vi "Generate Class and Subclasses.vi"(7 "Owning LVLib":refnum<vi>, 8 "Class Ref Map":T1, 9 "Class Name":string, 10 "Inheritance Map":T1, 11 "Base Class":refnum<vi>) -> (0 "Augmented Class Ref Map":T1, 2 "Reduced Inheritance Map":T1, 3 "Base Class Dup":refnum<vi>)   [LabVIEW 2013]
uses:
  <userlib>/ICON Technologies/ICON Maps/lvlib/Map.ctl
  <userlib>/ICON Technologies/ICON Maps/lvlib/_Polymorphic Instances/Map_Insert_Variant.vi
  <userlib>/ICON Technologies/ICON Maps/ICON Maps.lvlib
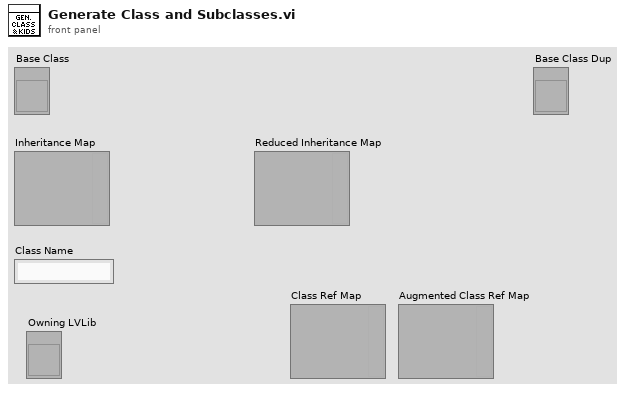
[diagram p1: front panel]
types:
  T1 = typedef "ICON Maps.lvlib/Map.ctl" = variant
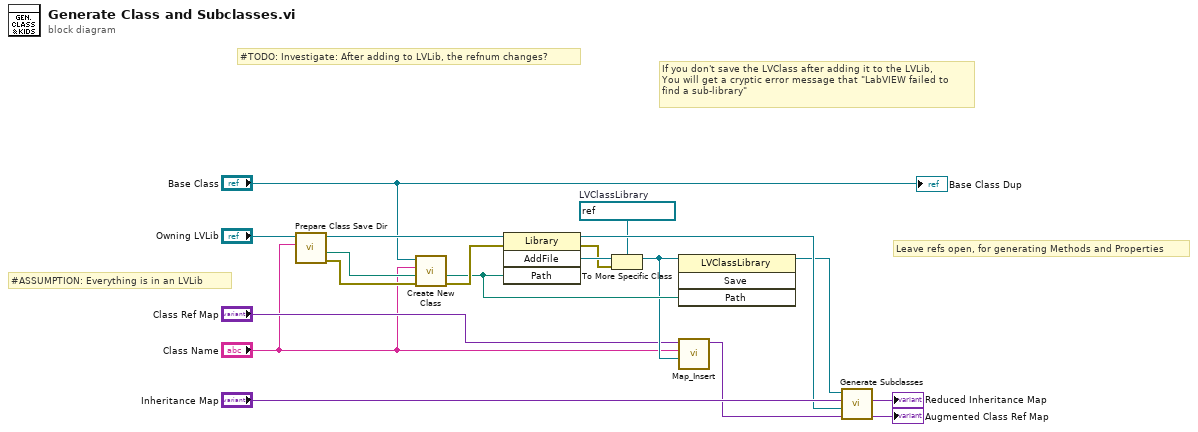
[diagram p0: block diagram]
diagram:
  w11 = refnum<vi> refnum  # LVClassLibrary
  # "Leave refs open, for generating Methods and Properties"
  # "#ASSUMPTION: Everything is in an LVLib"
  # "If you don't save the LVClass after adding it to the LVLib,\nYou will get a cryptic error message that \"LabVIEW failed to\nfind a sub-library\""
  # "#TODO: Investigate: After adding to LVLib, the refnum changes?"
  n1 = call "Prepare Class Save Dir.vi"("Class Name"="Class Name", "Owning LVLib"="Owning LVLib") -> ("Error Out"=w13:errorcluster, "Class Path"=w8:path, "Owning LVLib Dup"=w9:refnum<vi>)  [unwired: 7 in]
  n2 = call "Create New Class.vi"("Error In"=w13, "Class Path"=w8, "Class Name"="Class Name", "Base Class"="Base Class") -> ("Error Out"=w12:errorcluster, "Class Path Dup"=w7:path)  [unwired: 5 in, 1 out]
  n3 = invoke class="Library" method="AddFile"(reference=w9, error in=w12, "Path"=w7) -> (reference out=w16:refnum<vi>, error out=w14:errorcluster, "AddFile"=w17:refnum<vi>)  [unwired: 1 in, 1 out]
  n4 = To More Specific Class(target class=w11, reference=w17, error in=w14) -> (specific class reference=w6:refnum<vi>)  [unwired: 1 out]
  n5 = invoke class="LVClassLibrary" method="Save"(reference=w6, "Path"=w7) -> (reference out=w15:refnum<vi>)  [unwired: 2 in, 3 out]
  n6 = call-poly <userlib>:"Map_Insert.vi"("Value"=w6, "Key"="Class Name", "Map In"="Class Ref Map") -> ("Map Out"=w4:T1)  [unwired: 8 in]
  n7 = call "Generate Subclasses.vi"("Class Ref Map"=w4, "Owning LVLib"=w16, "Inheritance Map"="Inheritance Map", "Base Class"=w15) -> ("Augmented Class Ref Map"=→"Augmented Class Ref Map":T1, "Reduced Inheritance Map"=→"Reduced Inheritance Map":T1)  [unwired: 4 in, 2 out]
  "Base Class Dup" <- "Base Class"
